vi "Create Listbox Row.vi"(4 "swap new and old (F)":bool, 6 "override name":string, 7 "refresh symbol (Blank)":T2, 8 "change? (T)":bool=TRUE, 9 "new item":string, 10 "old item":string, 11 "refresh listbox":T1[](array[typedef])) -> (3 "refresh listbox out":T1[](array[typedef]))   [LabVIEW 2020, in "AIM ARINC 429 System Explorer.lvlib" / "Implementation.lvlib"]
uses:
  Implementation.lvlib
  Types/Refresh Symbols.ctl
  Types/Refresh Listbox.ctl
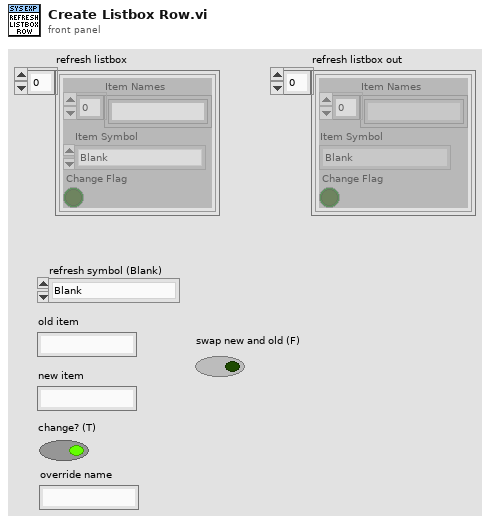
[diagram p1: front panel]
types:
  T1 = typedef "AIM ARINC 429 System Explorer.lvlib/Implementation.lvlib/Refresh Listbox.ctl" = cluster{"Item Names":string[], "Item Symbol":T2, "Change Flag":bool}
  T2 = typedef "AIM ARINC 429 System Explorer.lvlib/Implementation.lvlib/Refresh Symbols.ctl" = enum16{"Blank", "Port", "Incoming", "Outgoing", "Label", "Word", "Parameter", "ARINC-429", "Config Files", "Channel Spec", "Item"}
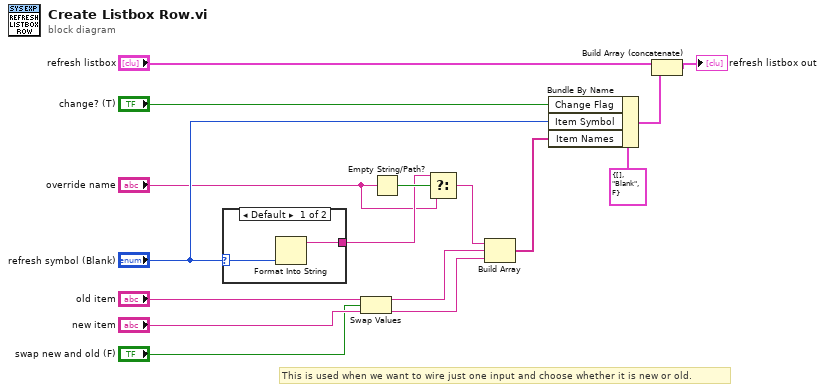
[diagram p0: block diagram]
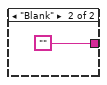
[diagram p2: hidden frame]
diagram:
  # "This is used when we want to wire just one input and choose whether it is new or old."
  n1 = case shown="Default" "refresh symbol (Blank)" {
    selector: "refresh symbol (Blank)" -> [w17 _]
    tunnel: [w18 ""] -> w13
    frame Default {
      n2 = Format Into String(w17) -> (resulting string=w18:string)  [unwired: 3 in, 1 out]
    }
    frame "Blank" {
    }
  }
  n3 = Swap Values(12:"old item", 13:"swap new and old (F)", 14:"new item") -> (1:w4:string, 3:w2:string)
  n4 = Empty String/Path?(string/path="override name") -> (empty?=w15:bool)
  n5 = Select(t=w13, s=w15, f="override name") -> (s? t:f=w14:string)
  n6 = Build Array(w14, w4, w2) -> (w6:string[])
  n7 = Bundle By Name(cluster=T1 {"Item Names"=[], "Item Symbol"=enum."Blank", "Change Flag"=FALSE} ("refresh listbox"), "Change Flag"="change? (T)", "Item Symbol"="refresh symbol (Blank)", "Item Names"=w6) -> (w10:T1)
  n8 = Build Array (concatenate)("refresh listbox", w10) -> (→"refresh listbox out":T1[])
